vi "StopStreaming.vi"(8 "error in (no error)":errorcluster, 11 "CameraDemo in":refnum<class "CameraDemo.lvclass">) -> (0 "error out":errorcluster, 3 "CameraDemo out":refnum<class "CameraDemo.lvclass">)   [LabVIEW 2020, in "CameraI2COUSB.lvlib" / "CameraDemo.lvclass"]
doc: "Stop streaming"
uses:
  CameraDemo.lvclass
  CameraDemo.lvclass/CameraDemo.ctl
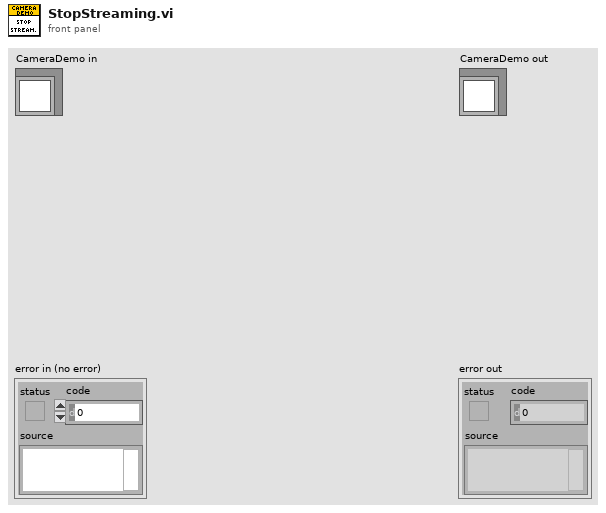
[diagram p1: front panel]
types:
  T1 = typedef "CameraI2COUSB.lvlib/CameraDemo.lvclass/StopStreamingEvnt.ctl" = refnum<user-event>
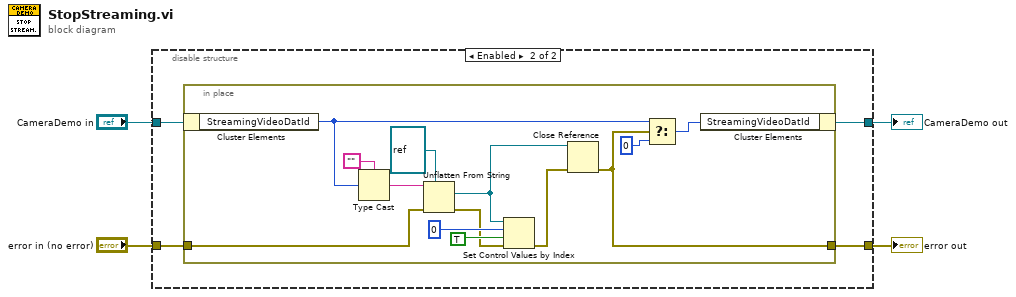
[diagram p0: block diagram]
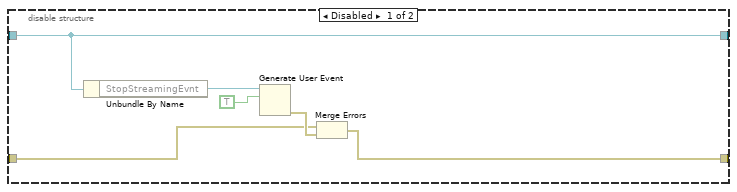
[diagram p2: hidden frame]
diagram:
  n1 = disable-structure shown="Enabled" {
    disable-tunnel: "CameraDemo in" -> [w5 w12]
    disable-tunnel: [w7 w14] -> w3
    disable-tunnel: "error in (no error)" -> [w6 w13]
    disable-tunnel: [w5 w11] -> w1
    frame Disabled {
      n2 = Unbundle By Name(w5) -> ("StopStreamingEvnt"=w10:T1)
      n3 = Generate User Event(user event=w10, event data cluster=TRUE ("event data")) -> (error out=w8:errorcluster)  [unwired: 2 in, 1 out]
      n4 = Merge Errors(w6, w8) -> (w7:errorcluster)
    }
    frame Enabled {
      n5 = in-place {
        in-place-border: [w15] -> w14
        in-place-border: w13 -> [w23]
        n6 = in-place-cluster #1(w12) -> ("StreamingVideoDatId"=w18:u32)
        n7 = Type Cast(type="", x=w18) -> (*(type *) &x=w24:string)
        n8 = Unflatten From String(type=refnum<vi> refnum ("type specifier VI Refnum (for type only)"), binary string=w24, error in (no error)=w23) -> (value=w19:refnum<vi>, error out=w22:errorcluster)  [unwired: 2 in, 1 out]
        n9 = Set Control Values by Index(0:w19, 1:0, 2:TRUE, 3:w22) -> (11:w20:errorcluster)
        n10 = Close Reference(reference=w19, error in (no error)=w20) -> (error out=w15:errorcluster)
        n11 = Select(t=w18, s=w15, f=u32 0) -> (s? t:f=w16:u32)
        n12 = in-place-cluster #1("StreamingVideoDatId"=w16) -> (w11:refnum<class "CameraDemo.lvclass">)
      }
    }
  }
  "error out" <- w3
  "CameraDemo out" <- w1
